vi "VALCCS_cal_vi_ver_1.5.vi"() -> ()   [LabVIEW 2019]
uses:
  <vilib>/ptbypt/NI_PtbyPt.lvlib
panel:
  out "Passenger Side Tyre":bool
  out "Driver Side Tyre":bool
  out "Total Axle Load (KG)":dbl
  out "Load Cell 3 Weight (KG)":dbl
  out "Weight 1":dbl
  out "Voltage 1":dbl
  out "Load Cell 3 Weight (KG)":dbl(graph)
  in  "stop":bool
  out "Load Cell 4 Weight (KG)":dbl
  out "Weight 2":dbl
  out "Voltage 2":dbl
  out "Load Cell 4  Weight (KG)":dbl(graph)
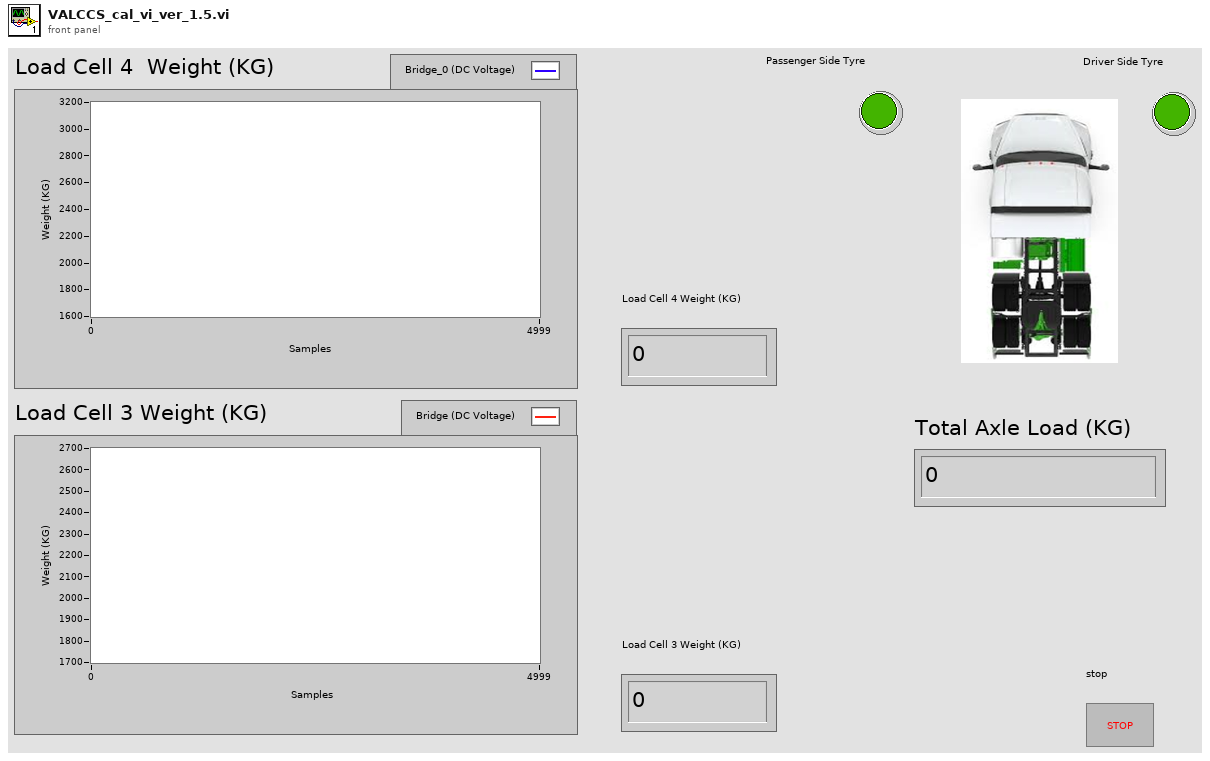
[diagram p1: front panel]
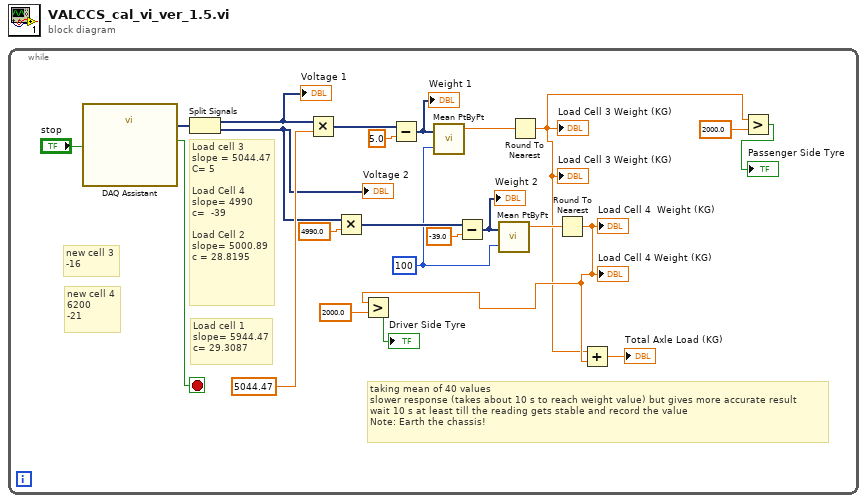
[diagram p0: block diagram]
diagram:
  n1 = while {
    stop <- w19 stop-if-true
    w9 = 100 ("sample length")
    # "new cell 3\n-16"
    # "new cell 4\n6200\n-21"
    # "taking mean of 40 values\nslower response (takes about 10 s to reach weight value) but gives more accurate result\nwait 10 s at least till the reading gets stable and record the value\nNote: Earth the chassis!"
    # "Load cell 1\nslope= 5944.47\nc= 29.3087"
    # "Load cell 3\nslope = 5044.47\nC= 5\n\nLoad Cell 4\nslope= 4990\nc=  -39\n\nLoad Cell 2\nslope= 5000.89\nc = 28.8195"
    n2 = call "DAQ Assistant"("stop (F)"="stop") -> ("data"=w18:dynamicdata, "stopped"=w19:bool)  [unwired: 15 in, 2 out]
    n3 = Split Signals(w18) -> (w14:dynamicdata, w13:dynamicdata)  [unwired: 2 in]
    "Voltage 2" <- w13
    "Voltage 1" <- w14
    n4 = Multiply(x=w14, y=5044.47) -> (x*y=w16:dynamicdata)
    n5 = Multiply(x=w13, y=4990.0) -> (x*y=w21:dynamicdata)
    n6 = Subtract(x=w16, y=5.0) -> (x-y=w12:dynamicdata)
    "Weight 1" <- w12
    n7 = call <vilib>:"Mean PtByPt.vi"("x"=w12, "sample length"=w9) -> ("mean"=w11:dbl)  [unwired: 2 in, 1 out]
    n8 = Subtract(x=w21, y=-39.0) -> (x-y=w10:dynamicdata)
    "Weight 2" <- w10
    n9 = call <vilib>:"Mean PtByPt.vi"("x"=w10, "sample length"=w9) -> ("mean"=w8:dbl)  [unwired: 2 in, 1 out]
    n10 = Round To Nearest(number=w11) -> (nearest integer value=w2:dbl)
    "Load Cell 3 Weight (KG)" <- w2
    "Load Cell 3 Weight (KG)" <- w2
    n11 = Round To Nearest(number=w8) -> (nearest integer value=w5:dbl)
    "Load Cell 4  Weight (KG)" <- w5
    "Load Cell 4 Weight (KG)" <- w5
    n12 = Greater?(x=w5, y=2000.0) -> (0:→"Driver Side Tyre":bool)
    n13 = Add(x=w2, y=w5) -> (x+y=→"Total Axle Load (KG)":dbl)
    n14 = Greater?(x=w2, y=2000.0) -> (0:→"Passenger Side Tyre":bool)
  }
